vi "convertForFPGA.vi"(8 "error in (no error)":errorcluster, 11 "Modbus in":refnum<class "Modbus.lvclass">) -> (0 "error out":errorcluster, 2 "Data":u16[](array[numeric]), 3 "Modbus out":refnum<class "Modbus.lvclass">)   [LabVIEW 2015, in "Modbus.lvclass"]
uses:
  Modbus.lvclass
  Modbus.lvclass/Modbus.ctl
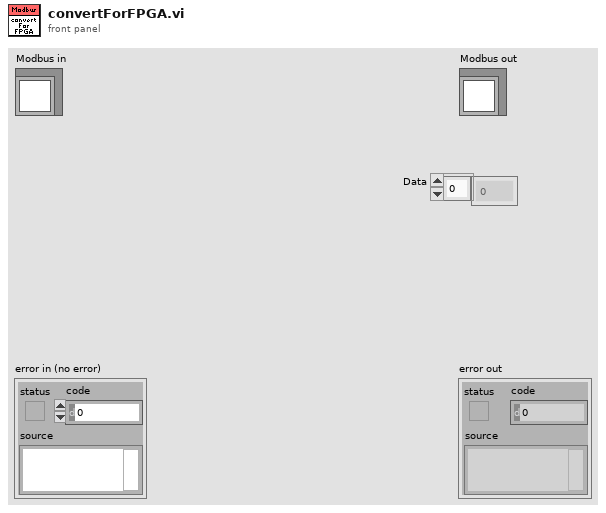
[diagram p1: front panel]
types:
  T1 = typedef "RTTypeDefs.lvlib/Frame.ctl" = cluster{"Data":u8[]}
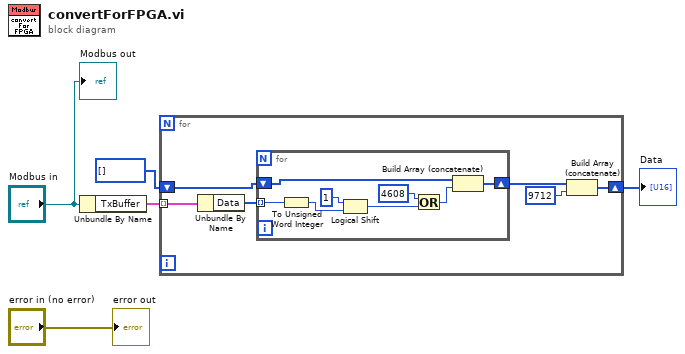
[diagram p0: block diagram]
diagram:
  n1 = Unbundle By Name("Modbus in") -> ("TxBuffer"=w5:T1[])
  n2 = for {
    tunnel: w5 -> [w11] mode=indexing
    shift-right: [w8] -> w2
    shift-left: u16[] [] -> [w10]
    n3 = Unbundle By Name(w11) -> ("Data"=w6:u8[])
    n4 = for {
      shift-right: [w18] -> w9
      shift-left: w10 -> [w19]
      tunnel: w6 -> [w12] mode=indexing
      n5 = To Unsigned Word Integer(number=w12) -> (unsigned 16bit integer=w17:u16)
      n6 = Logical Shift(y=i16 1, x=w17) -> (x << y=w15:u16)
      n7 = Or(x=u16 4608, y=w15) -> (x .or. y?=w13:u16)
      n8 = Build Array (concatenate)(w19, w13) -> (w18:u16[])
    }
    n9 = Build Array (concatenate)(w9, u16 9712 ("x")) -> (w8:u16[])
  }
  "Data" <- w2
  "error out" <- "error in (no error)"
  "Modbus out" <- "Modbus in"
